vi "read forward power dBm.vi"(3 "error in (no error)":errorcluster, 5 "VISA resource name":refnum<visa-resource-name>="GPIB0::12::INSTR") -> (0 "error out":errorcluster, 1 "forward power (dBm)":dbl, 2 "VISA resource name out":refnum<visa-resource-name>)   [LabVIEW 2009, in "MicrowaveAmplifier.lvlib"]
uses:
  MicrowaveAmplifier.lvlib
panel:
  out "read buffer":string
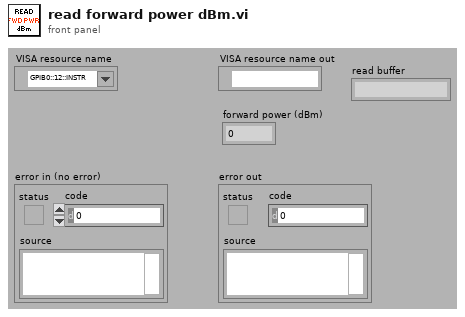
[diagram p1: front panel]
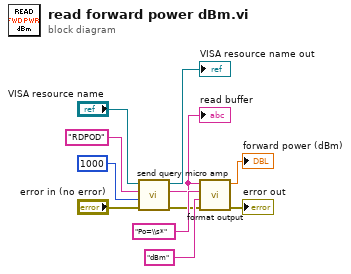
[diagram p0: block diagram]
diagram:
  n1 = call "send query micro amp.vi"("error in (no error)"="error in (no error)", "Bytes Count"=u32 1000 ("bytes to read (1000)"), "write buffer"="RDPOD", "VISA resource name"="VISA resource name") -> ("error out"=w2:errorcluster, "read buffer"=w1:string, "VISA resource name out"=→"VISA resource name out":refnum<visa-resource-name>)  [unwired: 5 in]
  "read buffer" <- w1
  n2 = call "format output.vi"("error in (no error)"=w2, "Search for String"="dBm" ("search string"), "Regular Expression"="Po=\\s*" ("search string"), "Input String"=w1) -> ("error out"=→"error out":errorcluster, "Output"=→"forward power (dBm)":dbl)  [unwired: 6 in]
